vi "get_filter_constant.vi"(8 "error in (no error)":errorcluster, 11 "VISA Refnum in":refnum<visa-resource-name>) -> (0 "error out":errorcluster, 2 "Filter constant":string, 3 "VISA Refnum out":refnum<visa-resource-name>)   [LabVIEW 2018]
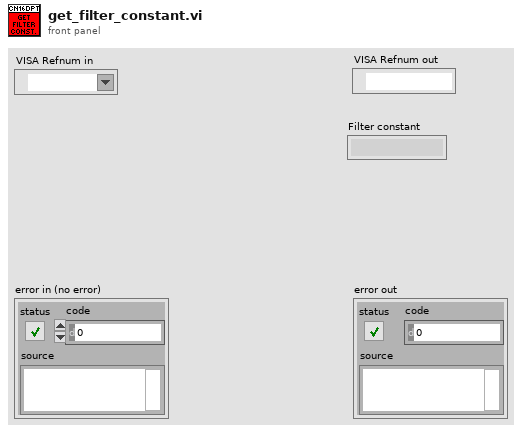
[diagram p1: front panel]
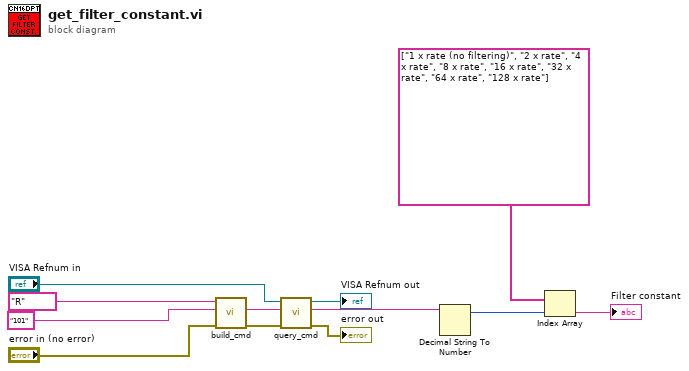
[diagram p0: block diagram]
diagram:
  n1 = call "build_cmd.vi"("error in (no error)"="error in (no error)", "Command ID"="101", "Command class"="R") -> ("error out"=w7:errorcluster, "Command"=w6:string)  [unwired: 7 in]
  n2 = call "query_cmd.vi"("error in (no error)"=w7, "Command"=w6, "VISA resource name"="VISA Refnum in") -> ("error out"=→"error out":errorcluster, "Response"=w3:string, "VISA resource name out"=→"VISA Refnum out":refnum<visa-resource-name>)  [unwired: 6 in]
  n3 = Decimal String To Number(string=w3) -> (offset past number=w4:i32)  [unwired: 2 in, 1 out]
  n4 = Index Array(array=string[] ["1 x rate (no filtering)", "2 x rate", "4 x rate", "8 x rate", "16 x rate", "32 x rate", "64 x rate", "128 x rate"], index=w4) -> (element=→"Filter constant":string)
